vi "Configure Library for Development.vi"(11 "library path":path) -> (0 "error out":errorcluster)   [LabVIEW 2017, in "Build Automation.lvlib"]
uses:
  Build Automation.lvlib
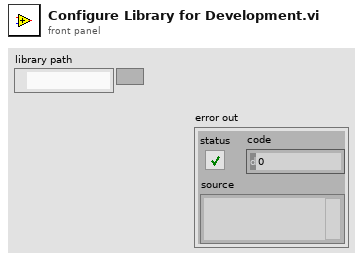
[diagram p1: front panel]
types:
  T1 = cluster{"Status Message":refnum<data-value>, "Progress":refnum<data-value>, "Stop":refnum<data-value>}
  T2 = enum16{"Share clones between instances", "Preallocate clone for each instance"}
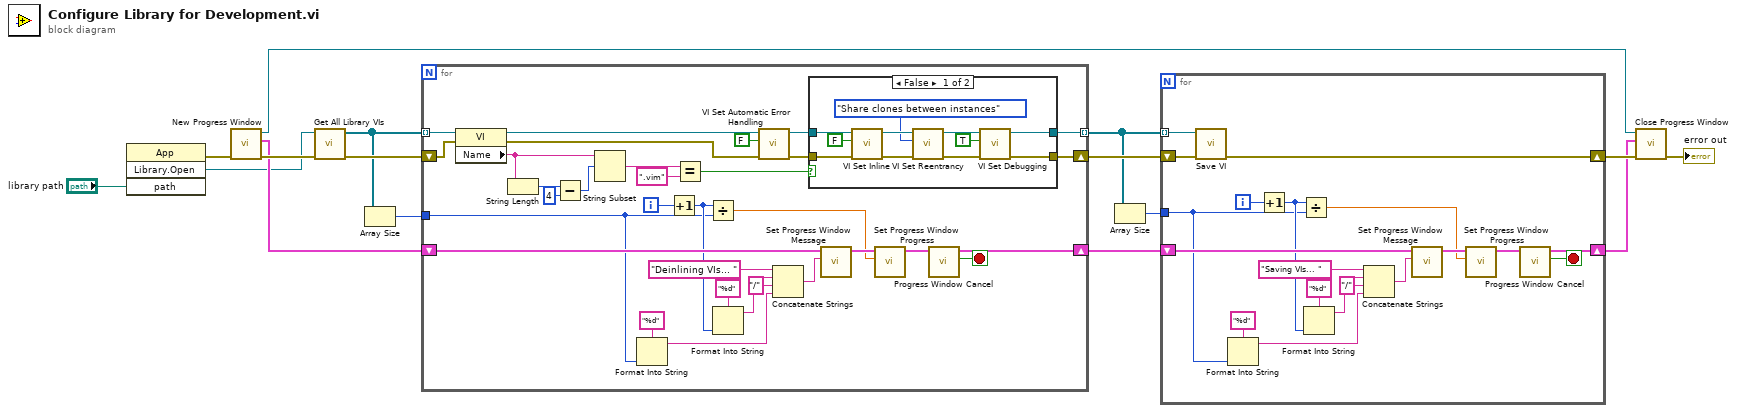
[diagram p0: block diagram]
diagram:
  n1 = invoke class="App" method="Library.Open"("path"="library path") -> (error out=w15:errorcluster, "Open Library"=w7:refnum<vi>)  [unwired: 3 in, 2 out]
  n2 = call "New Progress Window.vi"("error in (no error)"=w15) -> ("error out"=w9:errorcluster, "DVRs"=w8:T1, "VI refnum"=w12:refnum<vi>)  [unwired: 8 in]
  n3 = call "Get All Library VIs.vi"("error in (no error)"=w9, "library ref"=w7) -> ("error out"=w16:errorcluster, "vi refs"=w14:refnum<vi>[])  [unwired: 8 in]
  n4 = Array Size(array=w14) -> (size(s)=w13:i32)
  n5 = for {
    tunnel: w14 -> [w39] mode=indexing
    shift-right: [w46] -> w11
    shift-left: w16 -> [w38]
    tunnel: w13 -> [w22]
    shift-right: [w26] -> w10
    shift-left: w8 -> [w27]
    tunnel: [w47] -> w6 mode=indexing
    i -> [w48]
    stop <- w25 stop-if-true
    n6 = property class="VI"(reference=w39, error in=w38) -> (reference out=w19:refnum<vi>, error out=w21:errorcluster, "Name"=w45:string)
    n7 = String Length(string=w45) -> (length=w44:i32)
    n8 = Subtract(x=w44, y=4) -> (x-y=w40:i32)
    n9 = String Subset(string=w45, offset (0)=w40) -> (substring=w42:string)  [unwired: 1 in]
    n10 = Format Into String(format string="%d", w22) -> (resulting string=w29:string)  [unwired: 2 in, 1 out]
    n11 = Increment(x=w48) -> (x+1=w23:i32)
    n12 = Equal?(x=w42, y=".vim") -> (x = y?=w37:bool)
    n13 = Divide(x=w23, y=w22) -> (x/y=w24:dbl)
    n14 = Format Into String(format string="%d", w23) -> (resulting string=w34:string)  [unwired: 2 in, 1 out]
    n15 = call "VI Set Automatic Error Handling.vi"("error in (no error)"=w21, "Automatic Error Handling"=FALSE, "vi ref in"=w19) -> ("error out"=w20:errorcluster, "vi ref out"=w18:refnum<vi>)  [unwired: 7 in]
    n16 = Concatenate Strings("Deinlining VIs... " ("Status Message"), w34, "/" ("string"), w29) -> (w31:string)
    n17 = case shown="False" w37 {
      tunnel: [w49 w61] -> w47
      tunnel: [w52 w60] -> w46
      tunnel: w18 -> [w51 w61]
      tunnel: w20 -> [w50 w60]
      frame False {
        n18 = call "VI Set Inline.vi"("error in (no error)"=w50, "Inline VI"=FALSE, "vi ref in"=w51) -> ("error out"=w56:errorcluster, "vi ref out"=w57:refnum<vi>)  [unwired: 7 in]
        n19 = call "VI Set Reentrancy.vi"("error in (no error)"=w56, "Reentrancy Type"=T2."Share clones between instances", "vi ref in"=w57) -> ("error out"=w53:errorcluster, "vi ref out"=w54:refnum<vi>)  [unwired: 7 in]
        n20 = call "VI Set Debugging.vi"("error in (no error)"=w53, "Allow Debugging"=TRUE, "vi ref in"=w54) -> ("error out"=w52:errorcluster, "vi ref out"=w49:refnum<vi>)  [unwired: 7 in]
      }
      frame True {
      }
    }
    n21 = call "Set Progress Window Message.vi"("Status Message"=w31, "DVRs in"=w27) -> ("DVRs out"=w32:T1)  [unwired: 8 in, 1 out]
    n22 = call "Set Progress Window Progress.vi"("Progress"=w24, "DVRs in"=w32) -> ("DVRs out"=w28:T1)  [unwired: 8 in, 1 out]
    n23 = call "Progress Window Cancel.vi"("DVRs in"=w28) -> ("cancelled"=w25:bool, "DVRs out"=w26:T1)  [unwired: 8 in, 1 out]
  }
  n24 = Array Size(array=w6) -> (size(s)=w5:i32)
  n25 = for {
    shift-right: [w78] -> w4
    shift-left: w11 -> [w80]
    tunnel: w6 -> [w79] mode=indexing
    shift-right: [w63] -> w3
    shift-left: w10 -> [w67]
    tunnel: w5 -> [w65]
    i -> [w77]
    stop <- w62 stop-if-true
    n26 = call "Save VI.vi"("error in (no error)"=w80, "vi ref in"=w79) -> ("error out"=w78:errorcluster)  [unwired: 8 in, 1 out]
    n27 = Format Into String(format string="%d", w65) -> (resulting string=w69:string)  [unwired: 2 in, 1 out]
    n28 = Increment(x=w77) -> (x+1=w66:i32)
    n29 = Divide(x=w66, y=w65) -> (x/y=w64:dbl)
    n30 = Format Into String(format string="%d", w66) -> (resulting string=w74:string)  [unwired: 2 in, 1 out]
    n31 = Concatenate Strings("Saving VIs... " ("Status Message"), w74, "/" ("string"), w69) -> (w71:string)
    n32 = call "Set Progress Window Message.vi"("Status Message"=w71, "DVRs in"=w67) -> ("DVRs out"=w72:T1)  [unwired: 8 in, 1 out]
    n33 = call "Set Progress Window Progress.vi"("Progress"=w64, "DVRs in"=w72) -> ("DVRs out"=w68:T1)  [unwired: 8 in, 1 out]
    n34 = call "Progress Window Cancel.vi"("DVRs in"=w68) -> ("cancelled"=w62:bool, "DVRs out"=w63:T1)  [unwired: 8 in, 1 out]
  }
  n35 = call "Close Progress Window.vi"("error in (no error)"=w4, "DVRs in"=w3, "VI refnum"=w12) -> ("error out"=→"error out":errorcluster)  [unwired: 8 in]
